vi "valves_defcmds.vi"(0 "Input solution":dbl=1.0, 1 "Add to C":dbl, 2 "Rings to open":u32, 3 "error in":errorcluster, 4 "COM4 in":refnum<k24>) -> (5 "COM4 out":refnum<k24>, 6 "Commands out":T1, 7 "error out":errorcluster)   [LabVIEW 2018]
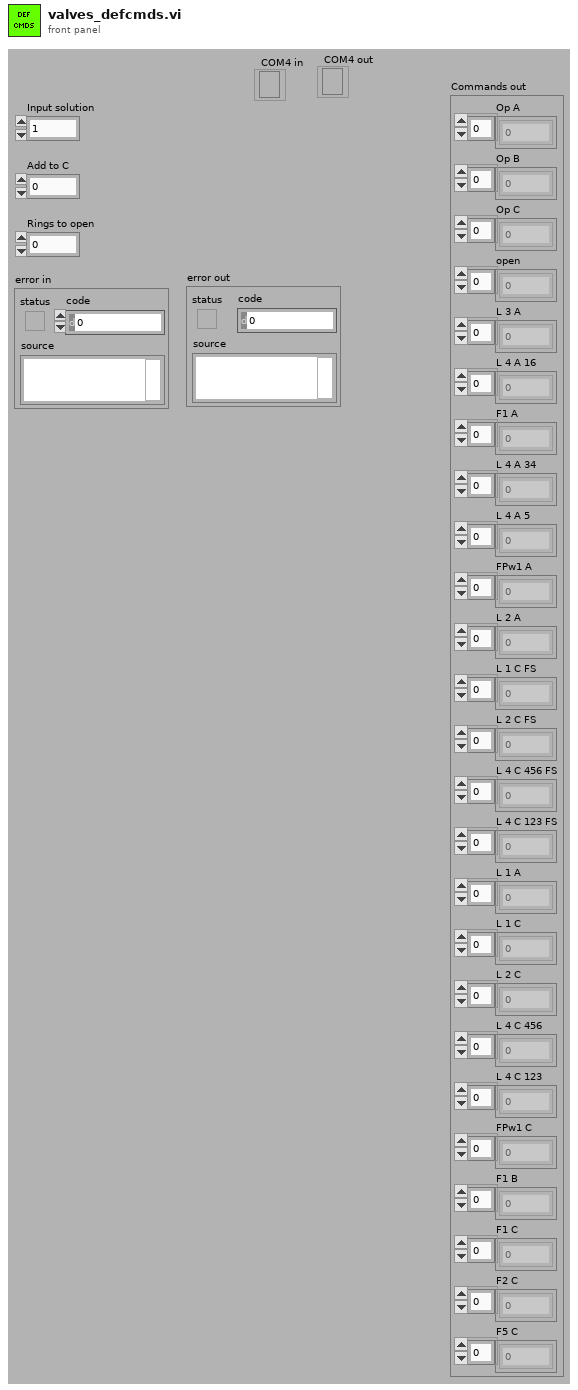
[diagram p1: front panel]
types:
  T1 = cluster{"Op A":u8[], "Op B":u8[], "Op C":u8[], "open":u8[], "L 3 A":u8[], "L 4 A 16":u8[], "F1 A":u8[], "L 4 A 34":u8[], "L 4 A 5":u8[], "FPw1 A":u8[], "L 2 A":u8[], "L 1 C FS":u8[], "L 2 C FS":u8[], "L 4 C 456 FS":u8[], "L 4 C 123 FS":u8[], "L 1 A":u8[], "L 1 C":u8[], "L 2 C":u8[], "L 4 C 456":u8[], "L 4 C 123":u8[], "FPw1 C":u8[], "F1 B":u8[], "F1 C":u8[], "F2 C":u8[], "F5 C":u8[]}
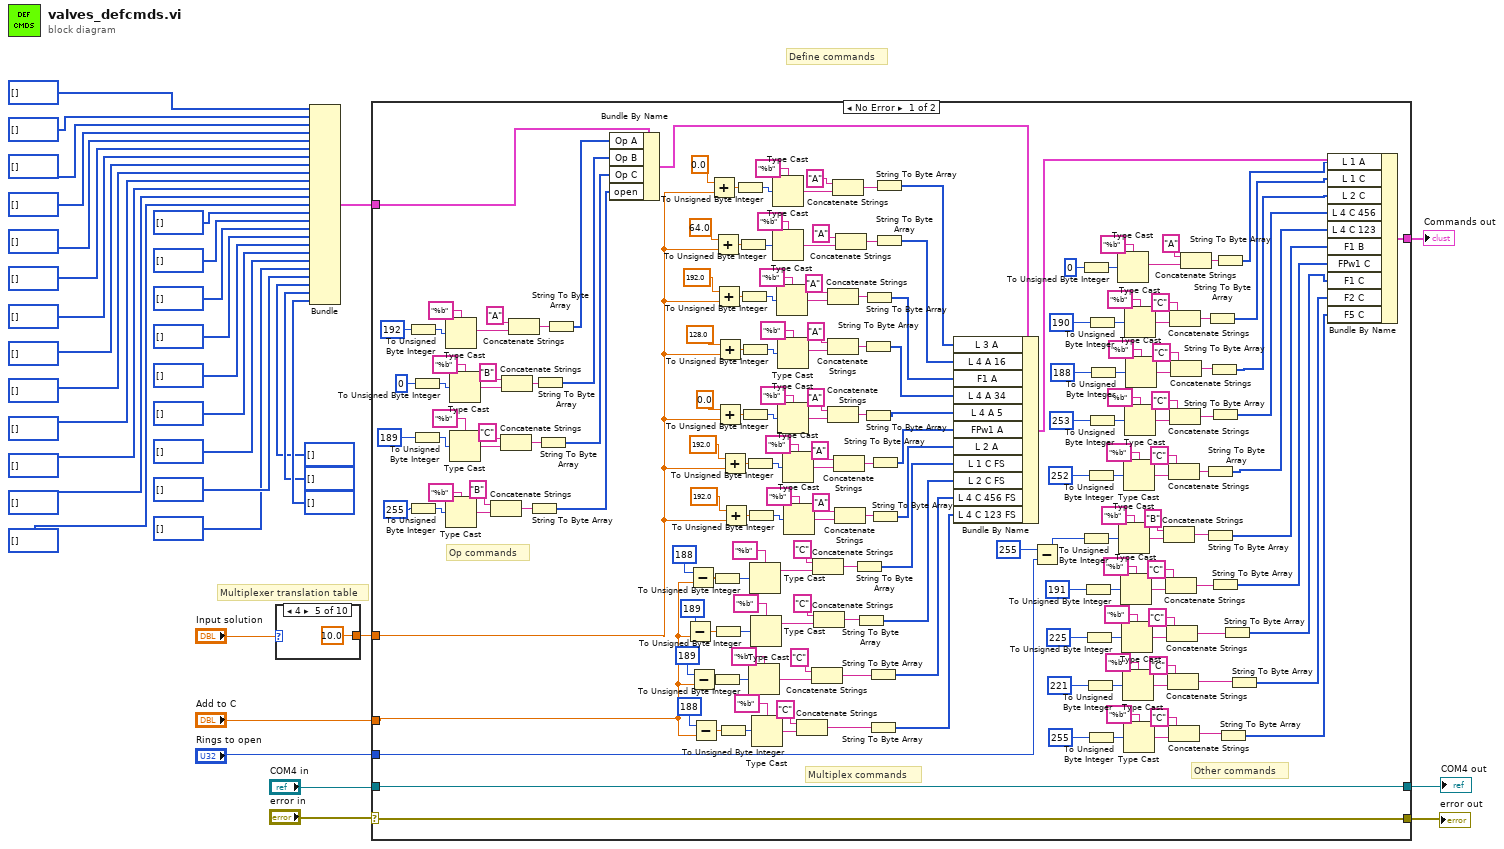
[diagram p0: block diagram]
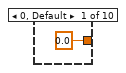
[diagram p3: hidden frame]
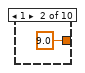
[diagram p4: hidden frame]
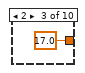
[diagram p5: hidden frame]
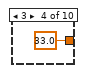
[diagram p6: hidden frame]
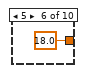
[diagram p7: hidden frame]
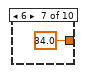
[diagram p8: hidden frame]
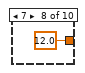
[diagram p9: hidden frame]
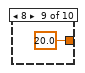
[diagram p10: hidden frame]
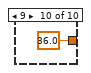
[diagram p11: hidden frame]
diagram:
  # "Define commands"
  # "Multiplexer translation table"
  n1 = case shown="4" "Input solution" {
    tunnel: [0.0 ("open flush") 9.0 ("open flush") 17.0 ("open flush") 33.0 ("open flush") 10.0 ("open flush") 18.0 ("open flush") 34.0 ("open flush") 12.0 ("open flush") 20.0 ("open flush") 36.0 ("open flush")] -> w31
    frame 0, Default {
    }
    frame 1 {
    }
    frame 2 {
    }
    frame 3 {
    }
    frame 4 {
    }
    frame 5 {
    }
    frame 6 {
    }
    frame 7 {
    }
    frame 8 {
    }
    frame 9 {
    }
  }
  n2 = Bundle("Op A"=u8[] [], "Op B"=u8[] [], "Op C"=u8[] [], "open"=u8[] [], "L 3 A"=u8[] [], "L 4 A 16"=u8[] [], "F1 A"=u8[] [], "L 4 A 34"=u8[] [], "L 4 A 5"=u8[] [], "FPw1 A"=u8[] [], "L 2 A"=u8[] [], "L 1 C FS"=u8[] [], "L 2 C FS"=u8[] [], "L 4 C 456 FS"=u8[] [], "L 4 C 123 FS"=u8[] [], "L 1 A"=u8[] [], "L 1 C"=u8[] [], "L 2 C"=u8[] [], "L 4 C 456"=u8[] [], "L 4 C 123"=u8[] [], "FPw1 C"=u8[] [], "F1 B"=u8[] [], "F1 C"=u8[] [], "F2 C"=u8[] [], "F5 C"=u8[] []) -> (w2:T1)  [unwired: 1 in]
  n3 = case shown="No Error" "error in" {
    selector: "error in" -> [w103 w243]
    tunnel: w31 -> [w241 _]
    tunnel: "Add to C" -> [w240 _]
    tunnel: "Rings to open" -> [w47 _]
    tunnel: [w103 w243] -> w35
    tunnel: "COM4 in" -> [w102 w244]
    tunnel: [w102 w244] -> w28
    tunnel: w2 -> [w100 w242]
    tunnel: [w49 w242] -> w1
    frame No Error {
      # "Other commands"
      # "Multiplex commands"
      # "Op commands"
      n4 = To Unsigned Byte Integer(number=u8 192) -> (unsigned 8bit integer=w225:u8)
      n5 = To Unsigned Byte Integer(number=u8 255) -> (unsigned 8bit integer=w224:u8)
      n6 = To Unsigned Byte Integer(number=u8 0) -> (unsigned 8bit integer=w228:u8)
      n7 = To Unsigned Byte Integer(number=u8 189) -> (unsigned 8bit integer=w233:u8)
      n8 = Type Cast(type="%b", x=w225) -> (*(type *) &x=w226:string)
      n9 = Type Cast(type="%b", x=w224) -> (*(type *) &x=w223:string)
      n10 = Type Cast(type="%b", x=w228) -> (*(type *) &x=w229:string)
      n11 = Type Cast(type="%b", x=w233) -> (*(type *) &x=w234:string)
      n12 = Concatenate Strings("B", w223) -> (w97:string)
      n13 = Concatenate Strings("C", w234) -> (w95:string)
      n14 = Concatenate Strings("B", w229) -> (w93:string)
      n15 = Concatenate Strings("A", w226) -> (w99:string)
      n16 = String To Byte Array(string=w97) -> (unsigned byte array=w96:u8[])
      n17 = String To Byte Array(string=w93) -> (unsigned byte array=w92:u8[])
      n18 = String To Byte Array(string=w95) -> (unsigned byte array=w94:u8[])
      n19 = String To Byte Array(string=w99) -> (unsigned byte array=w98:u8[])
      n20 = Bundle By Name(cluster=w100, "Op A"=w98, "Op B"=w92, "Op C"=w94, "open"=w96) -> (w105:T1)
      n21 = Subtract(x=u8 189 ("number"), y=w240) -> (x-y=w160:dbl)
      n22 = Subtract(x=u8 188 ("number"), y=w240) -> (x-y=w166:dbl)
      n23 = Subtract(x=u8 189 ("number"), y=w240) -> (x-y=w162:dbl)
      n24 = Subtract(x=u8 188 ("number"), y=w240) -> (x-y=w164:dbl)
      n25 = Add(x=0.0, y=w241) -> (x+y=w194:dbl)
      n26 = To Unsigned Byte Integer(number=w166) -> (unsigned 8bit integer=w168:u8)
      n27 = To Unsigned Byte Integer(number=w162) -> (unsigned 8bit integer=w176:u8)
      n28 = Add(x=64.0, y=w241) -> (x+y=w200:dbl)
      n29 = To Unsigned Byte Integer(number=w160) -> (unsigned 8bit integer=w172:u8)
      n30 = Add(x=192.0, y=w241) -> (x+y=w205:dbl)
      n31 = Add(x=128.0, y=w241) -> (x+y=w212:dbl)
      n32 = Add(x=0.0, y=w241) -> (x+y=w217:dbl)
      n33 = To Unsigned Byte Integer(number=w164) -> (unsigned 8bit integer=w180:u8)
      n34 = Add(x=192.0, y=w241) -> (x+y=w187:dbl)
      n35 = Add(x=192.0, y=w241) -> (x+y=w157:dbl)
      n36 = To Unsigned Byte Integer(number=w194) -> (unsigned 8bit integer=w190:u8)
      n37 = To Unsigned Byte Integer(number=w200) -> (unsigned 8bit integer=w196:u8)
      n38 = To Unsigned Byte Integer(number=w205) -> (unsigned 8bit integer=w202:u8)
      n39 = To Unsigned Byte Integer(number=w212) -> (unsigned 8bit integer=w208:u8)
      n40 = To Unsigned Byte Integer(number=w217) -> (unsigned 8bit integer=w213:u8)
      n41 = To Unsigned Byte Integer(number=w187) -> (unsigned 8bit integer=w184:u8)
      n42 = To Unsigned Byte Integer(number=w157) -> (unsigned 8bit integer=w154:u8)
      n43 = Type Cast(type="%b", x=w176) -> (*(type *) &x=w177:string)
      n44 = Type Cast(type="%b", x=w168) -> (*(type *) &x=w169:string)
      n45 = Type Cast(type="%b", x=w172) -> (*(type *) &x=w173:string)
      n46 = Type Cast(type="%b", x=w180) -> (*(type *) &x=w181:string)
      n47 = Type Cast(type="%b", x=w190) -> (*(type *) &x=w191:string)
      n48 = Type Cast(type="%b", x=w196) -> (*(type *) &x=w197:string)
      n49 = Type Cast(type="%b", x=w202) -> (*(type *) &x=w203:string)
      n50 = Type Cast(type="%b", x=w208) -> (*(type *) &x=w209:string)
      n51 = Type Cast(type="%b", x=w213) -> (*(type *) &x=w214:string)
      n52 = Type Cast(type="%b", x=w184) -> (*(type *) &x=w185:string)
      n53 = Type Cast(type="%b", x=w154) -> (*(type *) &x=w155:string)
      n54 = Concatenate Strings("C", w181) -> (w71:string)
      n55 = Concatenate Strings("C", w177) -> (w73:string)
      n56 = Concatenate Strings("C", w169) -> (w77:string)
      n57 = Concatenate Strings("C", w173) -> (w75:string)
      n58 = Concatenate Strings("A", w203) -> (w87:string)
      n59 = Concatenate Strings("A", w209) -> (w85:string)
      n60 = Concatenate Strings("A", w214) -> (w83:string)
      n61 = Concatenate Strings("A", w191) -> (w91:string)
      n62 = Concatenate Strings("A", w185) -> (w81:string)
      n63 = Concatenate Strings("A", w155) -> (w79:string)
      n64 = Concatenate Strings("A", w197) -> (w89:string)
      n65 = String To Byte Array(string=w77) -> (unsigned byte array=w76:u8[])
      n66 = String To Byte Array(string=w75) -> (unsigned byte array=w74:u8[])
      n67 = String To Byte Array(string=w85) -> (unsigned byte array=w84:u8[])
      n68 = String To Byte Array(string=w83) -> (unsigned byte array=w82:u8[])
      n69 = String To Byte Array(string=w87) -> (unsigned byte array=w86:u8[])
      n70 = String To Byte Array(string=w73) -> (unsigned byte array=w72:u8[])
      n71 = String To Byte Array(string=w71) -> (unsigned byte array=w70:u8[])
      n72 = String To Byte Array(string=w81) -> (unsigned byte array=w80:u8[])
      n73 = String To Byte Array(string=w79) -> (unsigned byte array=w78:u8[])
      n74 = String To Byte Array(string=w91) -> (unsigned byte array=w90:u8[])
      n75 = String To Byte Array(string=w89) -> (unsigned byte array=w88:u8[])
      n76 = Bundle By Name(cluster=w105, "L 3 A"=w90, "L 4 A 16"=w88, "F1 A"=w86, "L 4 A 34"=w84, "L 4 A 5"=w82, "FPw1 A"=w80, "L 2 A"=w78, "L 1 C FS"=w76, "L 2 C FS"=w74, "L 4 C 456 FS"=w72, "L 4 C 123 FS"=w70) -> (w104:T1)
      n77 = Subtract(x=u32 255, y=w47) -> (x-y=w46:u32)
      n78 = To Unsigned Byte Integer(number=u8 0) -> (unsigned 8bit integer=w145:u8)
      n79 = To Unsigned Byte Integer(number=w46) -> (unsigned 8bit integer=w150:u8)
      n80 = To Unsigned Byte Integer(number=u8 191) -> (unsigned 8bit integer=w143:u8)
      n81 = To Unsigned Byte Integer(number=u8 225) -> (unsigned 8bit integer=w138:u8)
      n82 = To Unsigned Byte Integer(number=u8 221) -> (unsigned 8bit integer=w133:u8)
      n83 = To Unsigned Byte Integer(number=u8 252) -> (unsigned 8bit integer=w108:u8)
      n84 = To Unsigned Byte Integer(number=u8 255) -> (unsigned 8bit integer=w129:u8)
      n85 = To Unsigned Byte Integer(number=u8 190) -> (unsigned 8bit integer=w123:u8)
      n86 = To Unsigned Byte Integer(number=u8 253) -> (unsigned 8bit integer=w114:u8)
      n87 = To Unsigned Byte Integer(number=u8 188) -> (unsigned 8bit integer=w118:u8)
      n88 = Type Cast(type="%b", x=w145) -> (*(type *) &x=w146:string)
      n89 = Type Cast(type="%b", x=w150) -> (*(type *) &x=w151:string)
      n90 = Type Cast(type="%b", x=w143) -> (*(type *) &x=w144:string)
      n91 = Type Cast(type="%b", x=w138) -> (*(type *) &x=w139:string)
      n92 = Type Cast(type="%b", x=w133) -> (*(type *) &x=w134:string)
      n93 = Type Cast(type="%b", x=w108) -> (*(type *) &x=w109:string)
      n94 = Type Cast(type="%b", x=w129) -> (*(type *) &x=w130:string)
      n95 = Type Cast(type="%b", x=w123) -> (*(type *) &x=w124:string)
      n96 = Type Cast(type="%b", x=w114) -> (*(type *) &x=w115:string)
      n97 = Type Cast(type="%b", x=w118) -> (*(type *) &x=w119:string)
      n98 = Concatenate Strings("B", w151) -> (w59:string)
      n99 = Concatenate Strings("C", w144) -> (w57:string)
      n100 = Concatenate Strings("C", w139) -> (w55:string)
      n101 = Concatenate Strings("C", w134) -> (w53:string)
      n102 = Concatenate Strings("C", w109) -> (w61:string)
      n103 = Concatenate Strings("C", w130) -> (w51:string)
      n104 = Concatenate Strings("C", w124) -> (w67:string)
      n105 = Concatenate Strings("C", w115) -> (w63:string)
      n106 = Concatenate Strings("C", w119) -> (w65:string)
      n107 = Concatenate Strings("A", w146) -> (w69:string)
      n108 = String To Byte Array(string=w61) -> (unsigned byte array=w60:u8[])
      n109 = String To Byte Array(string=w59) -> (unsigned byte array=w58:u8[])
      n110 = String To Byte Array(string=w67) -> (unsigned byte array=w66:u8[])
      n111 = String To Byte Array(string=w65) -> (unsigned byte array=w64:u8[])
      n112 = String To Byte Array(string=w63) -> (unsigned byte array=w62:u8[])
      n113 = String To Byte Array(string=w57) -> (unsigned byte array=w56:u8[])
      n114 = String To Byte Array(string=w69) -> (unsigned byte array=w68:u8[])
      n115 = String To Byte Array(string=w51) -> (unsigned byte array=w50:u8[])
      n116 = String To Byte Array(string=w55) -> (unsigned byte array=w54:u8[])
      n117 = String To Byte Array(string=w53) -> (unsigned byte array=w52:u8[])
      n118 = Bundle By Name(cluster=w104, "L 1 A"=w68, "L 1 C"=w66, "L 2 C"=w64, "L 4 C 456"=w62, "L 4 C 123"=w60, "F1 B"=w58, "FPw1 C"=w56, "F1 C"=w54, "F2 C"=w52, "F5 C"=w50) -> (w49:T1)
    }
    frame Error {
    }
  }
  "error out" <- w35
  "COM4 out" <- w28
  "Commands out" <- w1
